vi "Check_Point_Related.vi"(10 "Original Plots":dbl[](array[numeric]), 11 "Captured Plots":dbl[](array[numeric])) -> (3 "result":bool)   [LabVIEW 2012]
panel:
  out "counter":i32
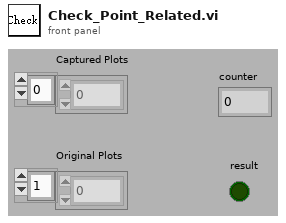
[diagram p1: front panel]
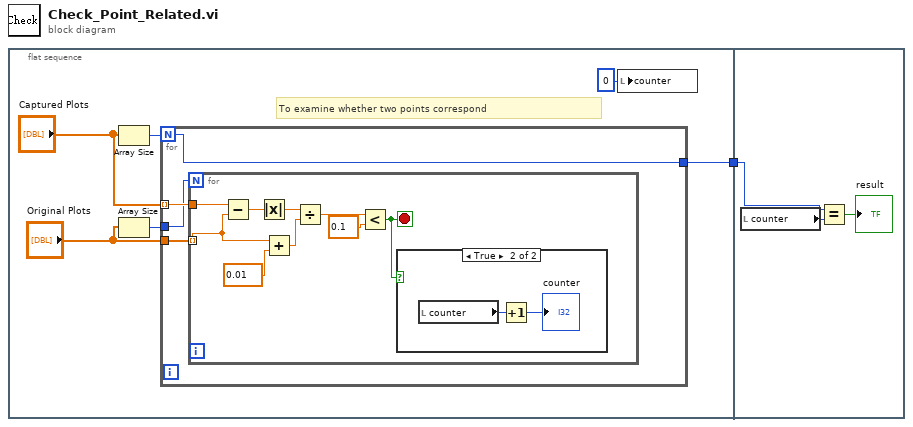
[diagram p0: block diagram]
diagram:
  n1 = flat-sequence {
    tunnel: [w3] -> w1
    tunnel: w1 -> [w23]
    frame #0 {
      # "To examine whether two points correspond"
      n2 = Array Size(array="Captured Plots") -> (size(s)=w7:i32)
      n3 = Array Size(array="Original Plots") -> (size(s)=w4:i32)
      n4 = for {
        N: w7 -> [w8]
        tunnel: "Captured Plots" -> [w11] mode=indexing
        tunnel: "Original Plots" -> [w10]
        tunnel: w4 -> [w9]
        tunnel: [w8] -> w3
        n5 = for {
          N: w9 -> [_]
          tunnel: w11 -> [w18]
          tunnel: w10 -> [w13] mode=indexing
          stop <- w19 stop-if-true
          n6 = Subtract(x=w18, y=w13) -> (x-y=w20:dbl)
          n7 = Absolute Value(x=w20) -> (abs(x)=w17:dbl)
          n8 = Add(x=w13, y=0.01) -> (x+y=w14:dbl)
          n9 = Divide(x=w17, y=w14) -> (x/y=w16:dbl)
          n10 = Less?(x=w16, y=0.1) -> (x < y?=w19:bool)
          n11 = case shown="True" w19 {
            frame False {
            }
            frame True {
              n12 = local read "counter"() -> (w22:i32)
              n13 = Increment(x=w22) -> (x+1=→"counter":i32)
            }
          }
        }
      }
      n14 = local write "counter"(0) -> ()
    }
    frame #1 {
      n15 = local read "counter"() -> (w24:i32)
      n16 = Equal?(x=w23, y=w24) -> (x = y?=→"result":bool)
    }
  }
